vi "Init.vi"() -> (0 "error out":errorcluster, 3 "Event Msg Type Strategy out":refnum<class "Event Msg Type Strategy.lvclass">)   [LabVIEW 2021, in "jettl.lvlib" / "Msg Type Strategy.lvlib" / "Event Msg Type Strategy.lvclass"]
uses:
  Event Msg Type Strategy.lvclass
  Msg Strategy/Msg Strategy.lvclass
  Event Msg Type Strategy.lvclass/Event Msg Type Strategy.ctl
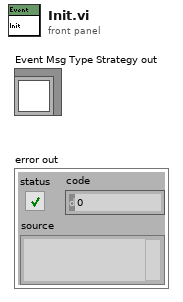
[diagram p1: front panel]
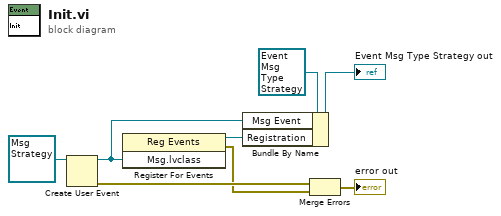
[diagram p0: block diagram]
diagram:
  n1 = Create User Event(user event datatype=refnum<class "Msg Strategy.lvclass"> refnum ("Msg.lvclass")) -> (user event=w4:refnum<user-event>, error out=w8:errorcluster)  [unwired: 1 in]
  n2 = register-events(w4) -> (reference out=w3:refnum<event-registration>, error out=w1:errorcluster)  [unwired: 2 in]
  n3 = Bundle By Name(cluster=refnum<class "Event Msg Type Strategy.lvclass"> refnum ("Event Msg Type Strategy out"), "Msg Event"=w4, "Registration"=w3) -> (→"Event Msg Type Strategy out":refnum<class "Event Msg Type Strategy.lvclass">)
  n4 = Merge Errors(w8, w1) -> (→"error out":errorcluster)
